vi "Convert Channel Bytes to Bit Array.vi"(0 "SRL Data":u8[][](array[numeric]) format="%02x", 1 "Cycle Mode In":bool) -> (4 "Write Data":u64[](array[numeric]) format="%016x")   [LabVIEW 2017, in "Host SRL.lvlib"]
uses:
  Host SRL.lvlib
panel:
  # "Non-Cycle Mode"
  # "Cycle Mode"
  # "Unused"
  # "#Cycle Commands"
  # "Channel"
  # "Ch-b0"
  # "DLY 1"
  # "CMD 1"
  # "DLY 2"
  # "CMD 2"
  # "DLY 3"
  # "CMD 3"
  # "CMD 4"
  # "DLY 4"
  # "Ch-b4"
  # "14-bit DAC Value"
  # "DAC-b0"
  # "DAC b4"
  # "DAC-b8"
  # "DAC-b12"
  # "DAC-b13"
  # "DLY 96"
  # "CMD 96"
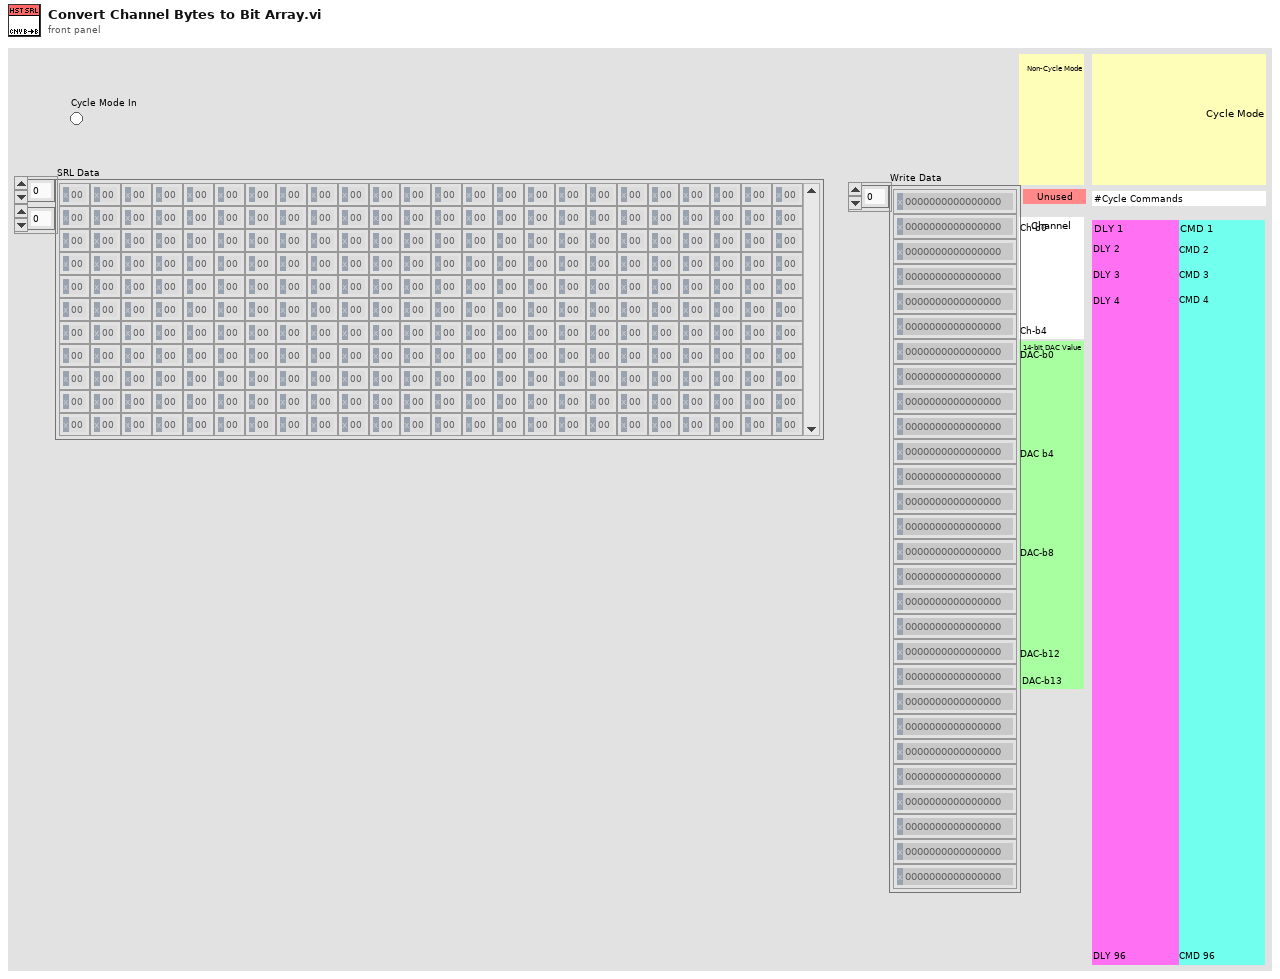
[diagram p1: front panel]
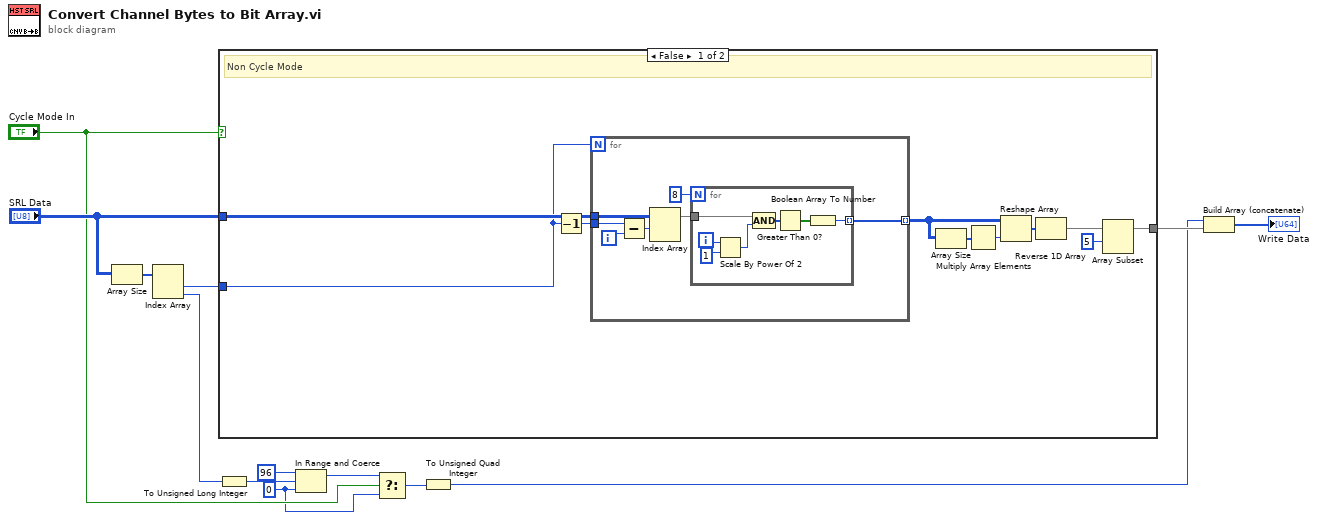
[diagram p0: block diagram]
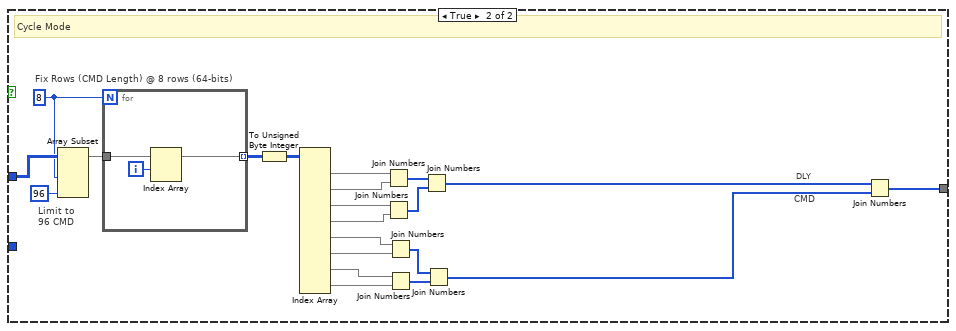
[diagram p2: hidden frame]
diagram:
  w4 = u32 0 ("lower limit")
  n1 = Array Size(array="SRL Data") -> (size(s)=w8:i32[])
  n2 = Index Array(array=w8) -> (element #1=w7:i32, element #2=w6:i32)  [unwired: 2 in]
  n3 = case shown="False" "Cycle Mode In" {
    tunnel: "SRL Data" -> [w16 w48]
    tunnel: [w18 w40] -> w10
    tunnel: w7 -> [w14 _]
    frame False {
      # "Non Cycle Mode"
      n4 = Decrement(x=w14) -> (x-1=w19:i32)
      n5 = for {
        N: w14 -> [_]
        tunnel: w16 -> [w28]
        tunnel: [w29] -> w23 mode=indexing
        tunnel: w19 -> [w24]
        i -> [w26]
        n6 = Subtract(x=w24, y=w26) -> (x-y=w25:i32)
        n7 = Index Array(array=w28, index (row)=w25) -> (element=w27:u8[])  [unwired: 1 in]
        n8 = for {
          N: 8 -> [_]
          tunnel: w27 -> [w33]
          tunnel: [w32] -> w29 mode=indexing
          i -> [w35]
          n9 = Scale By Power Of 2(n=w35, x=u8 1) -> (x*2^n=w36:u8)
          n10 = Compound Arithmetic op=AND(w33, w36) -> (w37:u8[])
          n11 = Greater Than 0?(x=w37) -> (x > 0?=w31:bool[])
          n12 = Boolean Array To Number(Boolean array=w31) -> (number=w32:u64)
        }
      }
      n13 = Array Size(array=w23) -> (size(s)=w22:i32[])
      n14 = Multiply Array Elements(1:w22) -> (0:w21:i32)
      n15 = Reshape Array(w23, w21) -> (w20:u64[])
      n16 = Reverse 1D Array(array=w20) -> (reversed array=w15:u64[])
      n17 = Array Subset(array=w15, index=5) -> (w18:u64[])  [unwired: 1 in]
    }
    frame True {
      w46 = 8
      # "CMD"
      # "DLY"
      # "Limit to\n96 CMD"
      # "Fix Rows (CMD Length) @ 8 rows (64-bits)"
      # "Cycle Mode"
      n18 = Array Subset(array=w48, length (row)=w46, length (col)=96 ("length")) -> (w47:u8[][])  [unwired: 2 in]
      n19 = for {
        N: w46 -> [_]
        tunnel: w47 -> [w61]
        tunnel: [w59] -> w49 mode=indexing
        i -> [w60]
        n20 = Index Array(array=w61, index (row)=w60) -> (element=w59:u8[])  [unwired: 1 in]
      }
      n21 = To Unsigned Byte Integer(number=w49) -> (unsigned 8bit integer=w52:u8[][])
      n22 = Index Array(array=w52) -> (element #1=w58:u8[], element #2=w57:u8[], element #3=w56:u8[], element #4=w55:u8[], element #5=w51:u8[], element #6=w44:u8[], element #7=w43:u8[], element #8=w42:u8[])  [unwired: 16 in]
      n23 = Join Numbers(hi=w58, lo=w57) -> ((hi.lo)=w54:u16[])
      n24 = Join Numbers(hi=w56, lo=w55) -> ((hi.lo)=w53:u16[])
      n25 = Join Numbers(hi=w51, lo=w44) -> ((hi.lo)=w50:u16[])
      n26 = Join Numbers(hi=w43, lo=w42) -> ((hi.lo)=w41:u16[])
      n27 = Join Numbers(hi=w54, lo=w53) -> ((hi.lo)=w38:u32[])
      n28 = Join Numbers(hi=w50, lo=w41) -> ((hi.lo)=w39:u32[])
      n29 = Join Numbers(hi=w38, lo=w39) -> ((hi.lo)=w40:u64[])
    }
  }
  n30 = To Unsigned Long Integer(number=w6) -> (unsigned 32bit integer=w11:u32)
  n31 = In Range and Coerce(upper limit=u32 96, x=w11, lower limit=w4) -> (coerced(x)=w3:u32)  [unwired: 1 out]
  n32 = Select(t=w3, s="Cycle Mode In", f=w4) -> (s? t:f=w2:u32)
  n33 = To Unsigned Quad Integer(1:w2) -> (0:w1:u64)
  n34 = Build Array (concatenate)(w1, w10) -> (→"Write Data":u64[])
